vi "Delete Services Table.vi"(8 "error in (no error)":errorcluster, 11 "Manejo Turnos in":refnum<class "Manejo Turnos.lvclass">) -> (0 "error out":errorcluster, 3 "Manejo Turnos out":refnum<class "Manejo Turnos.lvclass">)   [LabVIEW 2020, in "Manejo Turnos.lvlib" / "Manejo Turnos.lvclass"]
uses:
  Manejo Turnos.lvclass
  Manejo Turnos.lvclass/Manejo Turnos.ctl
  <vilib>/drjdpowell/SQLite Library/SQL Connection/Open (path).vi
  <vilib>/drjdpowell/SQLite Library/SQL Connection/Open (string).vi
  <vilib>/AdvancedString/Path To Command Line String.vi
  <vilib>/drjdpowell/SQLite Library/SQL Connection/Execute SQL (No results).vi
  <vilib>/drjdpowell/SQLite Library/SQL Connection/Connection.lvclass
  <vilib>/drjdpowell/SQLite Library/SQLite.lvlib
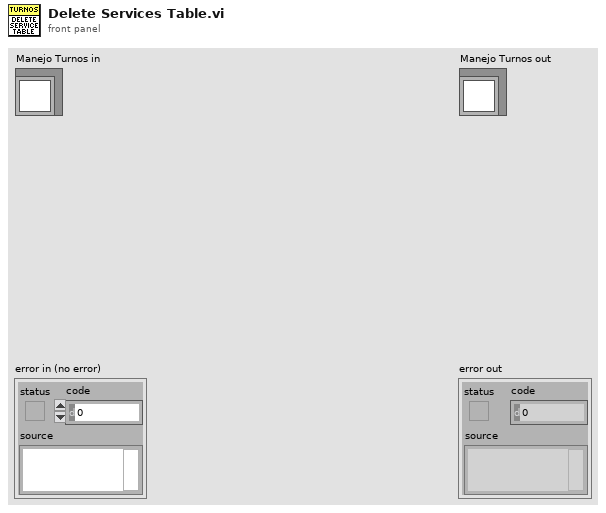
[diagram p1: front panel]
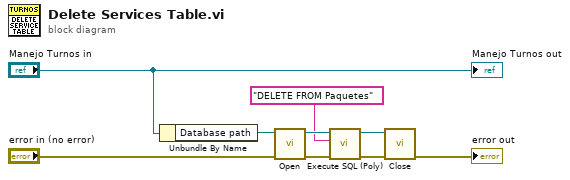
[diagram p0: block diagram]
diagram:
  n1 = Unbundle By Name("Manejo Turnos in") -> ("Database path"=w4:path)
  n2 = call-poly <vilib>:"Open.vi"("error in (no error)"="error in (no error)", "db file"=w4) -> ("error out"=w9:errorcluster, "SQLite Connection"=w3:refnum<class "Connection.lvclass">)  [unwired: 8 in]
  n3 = call-poly <vilib>:"Execute SQL (Poly).vi"("error in (no error)"=w9, "SQL"="DELETE FROM Paquetes", "SQLite Connection in"=w3) -> ("error out"=w8:errorcluster, "SQLite Connection"=w2:refnum<class "Connection.lvclass">)  [unwired: 7 in]
  n4 = call-dynamic "Close.vi"("error in (no error)"=w8, "SQLite Connection in"=w2) -> ("error out"=→"error out":errorcluster)  [unwired: 9 in]
  "Manejo Turnos out" <- "Manejo Turnos in"
